vi "XY_translation_Z_rotation.vi"() -> ()   [LabVIEW 2021]
uses:
  <instrlib>/Xbox-One-Controller/Private/Type Defs/Indicators/Controller.ctl
  <instrlib>/Xbox-One-Controller/Private/Type Defs/Indicators/A.ctl
  <instrlib>/Xbox-One-Controller/Private/Type Defs/Indicators/B.ctl
  <instrlib>/Xbox-One-Controller/Private/Type Defs/Indicators/X.ctl
  <instrlib>/Xbox-One-Controller/Private/Type Defs/Indicators/Y.ctl
  <instrlib>/Xbox-One-Controller/Private/Type Defs/Indicators/Left Bumper.ctl
  <instrlib>/Xbox-One-Controller/Private/Type Defs/Indicators/Right Bumper.ctl
  <instrlib>/Xbox-One-Controller/Private/Type Defs/Indicators/View.ctl
  <instrlib>/Xbox-One-Controller/Private/Type Defs/Indicators/Menu.ctl
  <instrlib>/Xbox-One-Controller/Private/Type Defs/Indicators/Thumbstick_Analog.ctl
  <instrlib>/Xbox-One-Controller/Private/Type Defs/Indicators/Slider.ctl
  <instrlib>/Xbox-One-Controller/Private/Type Defs/Indicators/DPad.ctl
  C:/Program Files (x86)/Control/SC3U.dll
  <vilib>/Platform/TimedLoop/XDataNode/timing_clust.ctl
  <vilib>/Platform/TimedLoop/XDataNode/nitl_modes.ctl
  <vilib>/Platform/TimedLoop/XDataNode/wakeup.ctl
  <instrlib>/Xbox-One-Controller/Public/Open First Controller.vi
  <vilib>/Platform/TimedLoop/XDataNode/XDataNode.xnode
  <vilib>/Platform/TimedLoop/XDataNode/XDNodeRunTimeDep.lvlib
  <instrlib>/Xbox-One-Controller/LMH-Xbox-One-Controller.lvlib
panel:
  out "Pos X":dbl
  out "Pos Z":dbl
  in  "Com Close 3":bool
  in  "Displace Z":i64
  out "Pos Y mm":dbl
  in  "Displace Y":i64
  in  "Com Close 2":bool
  in  "Stop Button":bool
  out "Controller":T1={"A Button"=FALSE, "B Button"=FALSE, "X Button"=FALSE, "Y Button"=FALSE, "Left Bumper"=FALSE, "Right Bumper"=FALSE, "View Button"=FALSE, "Menu Button"=FALSE, "Left Stick"={[], []}, "Right Stick"={[], []}, "Trigger"=0, "D-Pad"=5} {"Trigger" scale=32767.0..-32768.0}
  in  "SC3U":refnum<k24>(container)
  in  "Com Close":bool
  in  "Displace X":i64
  out "ConnectStatus":bool
  out "ComUsing":i16
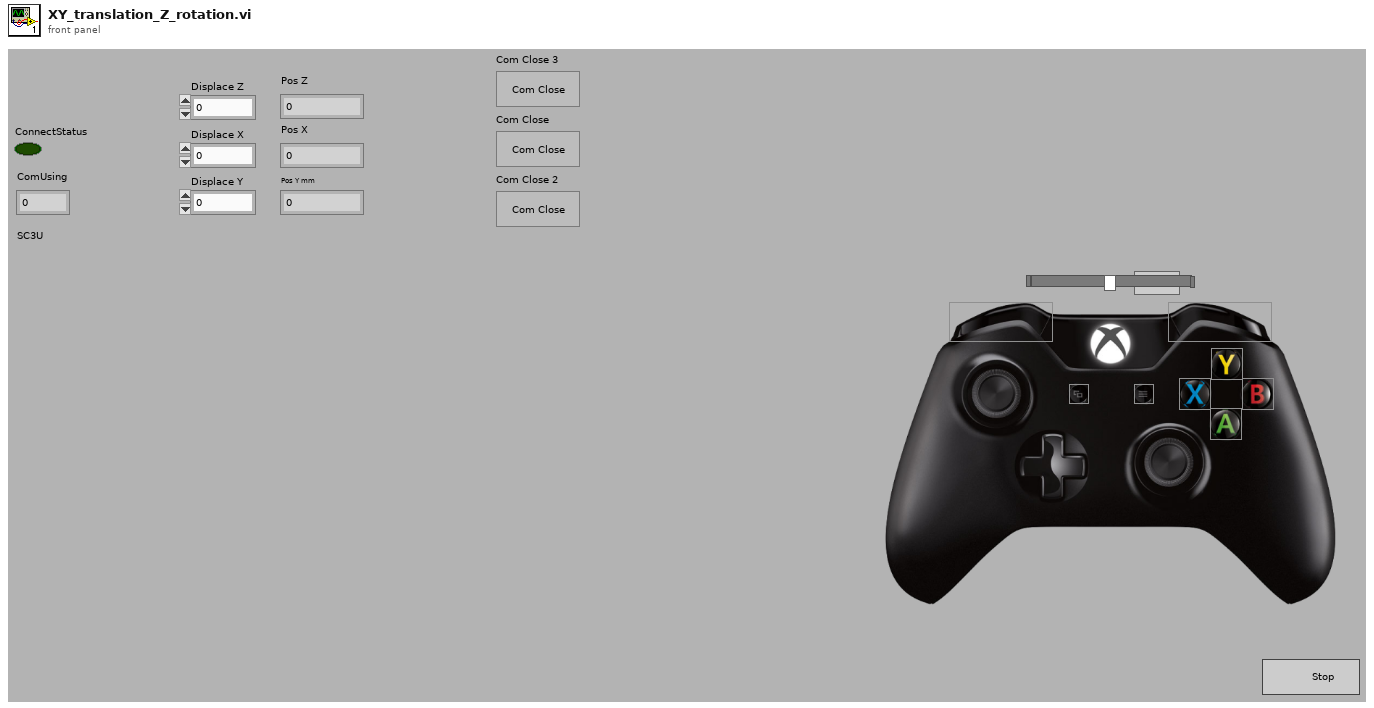
[diagram p1: front panel]
types:
  T1 = typedef "LMH-Xbox-One-Controller.lvlib/Controller.ctl" = cluster{"A Button":T2, "B Button":T3, "X Button":T4, "Y Button":T5, "Left Bumper":T6, "Right Bumper":T7, "View Button":T8, "Menu Button":T9, "Left Stick":T10, "Right Stick":T10, "Trigger":T11, "D-Pad":T12}
  T2 = typedef "LMH-Xbox-One-Controller.lvlib/A.ctl" = bool
  T3 = typedef "LMH-Xbox-One-Controller.lvlib/B.ctl" = bool
  T4 = typedef "LMH-Xbox-One-Controller.lvlib/X.ctl" = bool
  T5 = typedef "LMH-Xbox-One-Controller.lvlib/Y.ctl" = bool
  T6 = typedef "LMH-Xbox-One-Controller.lvlib/Left Bumper.ctl" = bool
  T7 = typedef "LMH-Xbox-One-Controller.lvlib/Right Bumper.ctl" = bool
  T8 = typedef "LMH-Xbox-One-Controller.lvlib/View.ctl" = bool
  T9 = typedef "LMH-Xbox-One-Controller.lvlib/Menu.ctl" = bool
  T10 = typedef "LMH-Xbox-One-Controller.lvlib/Thumbstick_Analog.ctl" = cluster{i32[], i32[]}
  T11 = typedef "LMH-Xbox-One-Controller.lvlib/Slider.ctl" = i32
  T12 = typedef "LMH-Xbox-One-Controller.lvlib/DPad.ctl" = u16
  T13 = typedef "XDNodeRunTimeDep.lvlib/timing_clust.ctl" = cluster{"Expected End [f-1]":u64, "Actual End [f-1]":u64, "Finished Late? [f-1]":bool, "Expected End [i-1]":u64, "Actual End [i-1]":u64, "Finished Late? [i-1]":bool, "Expected Start [i]":u64, "Actual Start [i]":u64, "Expected Start [f]":u64, "Actual Start [f]":u64, "Source Name":string, "Structure Name":string, "Period":i64, "Deadline":i64, "Offset":i64, "Start":i64, "Priority":i32, "Timeout":i32, "Mode":T14, "Wakeup Reason":T15, "Error":errorcluster, "Source Type":string, "Secondary Source Type":string, "Global End Time":u64, "Global Start Time":u64, "Frame Duration":u64, "Iteration Duration":u64, "Assigned CPU":i32, "I/O Scan Engine Mode":u32}
  T14 = typedef "XDNodeRunTimeDep.lvlib/nitl_modes.ctl" = enum32{"No Change", "Process missed periods, maintain original phase", "Discard missed periods, maintain original phase", "Process missed periods, ignore original phase", "Discard missed periods, ignore original phase"}
  T15 = typedef "XDNodeRunTimeDep.lvlib/wakeup.ctl" = enum32{"Normal", "Aborted", "Asynchronous wakeup", "Timing source error", "Timed loop error", "Timeout"}
  T16 = typedef "LMH-Xbox-One-Controller.lvlib/Xbox One Controller Ref.ctl" = cluster{"Controller Ref":refnum<k1>, "Event Refnum":refnum<event-registration>, "Worker Ref":refnum<vi>}
  T17 = typedef "LMH-Xbox-One-Controller.lvlib/All Axis Data.ctl" = cluster{"Left Stick":cluster{"X Axis":i32, "Y Axis":i32}, "Right Stick":cluster{"X Axis":i32, "Y Axis":i32}, "Triggers":i32, "D-Pad":T18}
  T18 = typedef "LMH-Xbox-One-Controller.lvlib/DPad Enum.ctl" = enum16{"Idle", "Up", "Up / Right", "Right", "Down / Right", "Down", "Down / Left", "Left", "Up / Left"}
  T19 = typedef "LMH-Xbox-One-Controller.lvlib/All Buttons Visual.ctl" = cluster{"A":T2, "B":T3, "X":T4, "Y":T5, "Left Bumper":T6, "Right Bumper":T7, "View Button":T8, "Menu Button":T9, "Left Stick":T20, "Right Stick":T20}
  T20 = typedef "LMH-Xbox-One-Controller.lvlib/Thumbstick.ctl" = bool
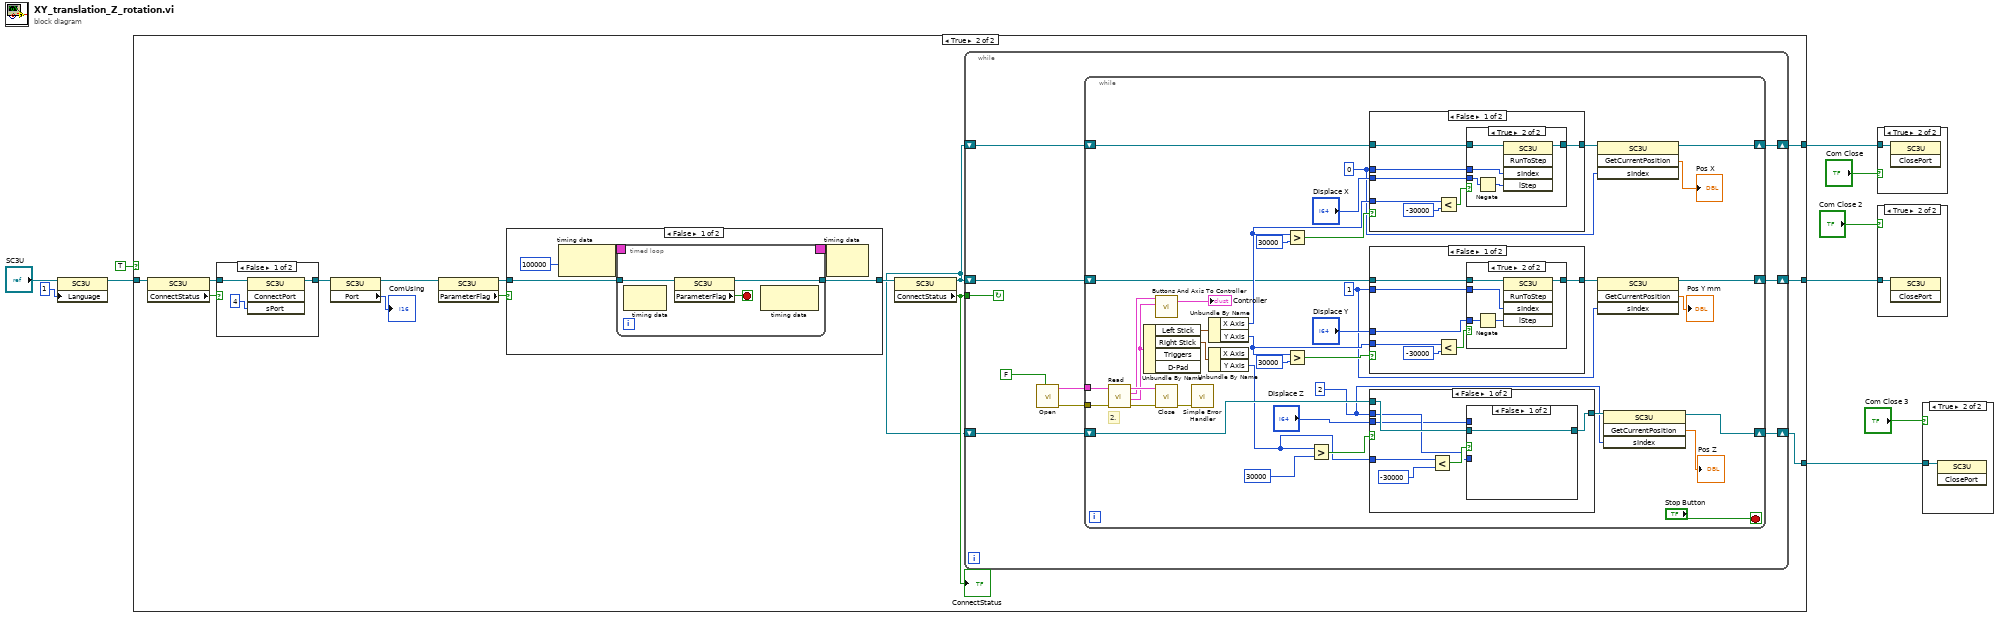
[diagram p0: block diagram]
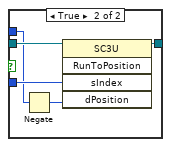
[diagram p6: hidden frame]
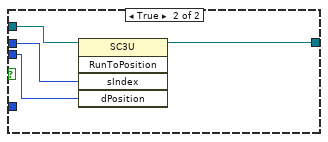
[diagram p7: hidden frame]
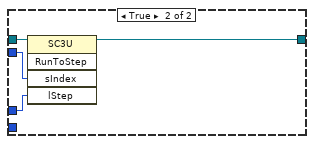
[diagram p9: hidden frame]
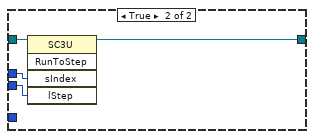
[diagram p11: hidden frame]
diagram:
  n1 = property class="SC3U"(reference="SC3U", "Language"=i16 1 ("intLanguage")) -> (reference out=w3:refnum<k24>)  [unwired: 1 in, 1 out]
  n2 = case shown="True" TRUE {
    tunnel: [_ w14] -> w6
    tunnel: w3 -> [_ w23]
    tunnel: [_ w13] -> w4
    tunnel: [_ w11] -> w1
    frame False {
    }
    frame True {
      n3 = property class="SC3U"(reference=w23) -> (reference out=w22:refnum<k24>, "ConnectStatus"=w21:bool)  [unwired: 1 in, 1 out]
      n4 = case shown="False" w21 {
        tunnel: w22 -> [w141 w142]
        tunnel: [w140 w142] -> w20
        frame False {
          n5 = invoke class="SC3U" method="ConnectPort"(reference=w141, "sPort"=i16 4 ("ComUsing")) -> (reference out=w140:refnum<k24>)  [unwired: 2 in, 3 out]
        }
        frame True {
        }
      }
      n6 = property class="SC3U"(reference=w20) -> (reference out=w18:refnum<k24>, "Port"=→"ComUsing":i16)  [unwired: 1 in, 1 out]
      n7 = property class="SC3U"(reference=w18) -> (reference out=w17:refnum<k24>, "ParameterFlag"=w16:bool)  [unwired: 1 in, 1 out]
      n8 = case shown="False" w16 {
        tunnel: w17 -> [w125 w138]
        tunnel: [w124 w138] -> w24
        frame False {
          n9 = node-c288(i64 100000 ("周期")) -> (w128:T13)
          n10 = timed-loop {
            timing: w128 -> [_]
            timing-out: [_] -> w127
            tunnel: w125 -> [w131]
            tunnel: [w130] -> w124
            stop <- w129 stop-if-true
            n11 = node-c288() -> ()  [unwired: 1 in, 1 out]
            n12 = property class="SC3U"(reference=w131) -> (reference out=w130:refnum<k24>, "ParameterFlag"=w129:bool)  [unwired: 1 in, 1 out]
            n13 = node-c288() -> ()  [unwired: 1 in, 1 out]
          }
          n14 = node-c288(w127) -> ()  [unwired: 1 out]
        }
        frame True {
        }
      }
      n15 = property class="SC3U"(reference=w24) -> (reference out=w12:refnum<k24>, "ConnectStatus"=w15:bool)  [unwired: 1 in, 1 out]
      "ConnectStatus" <- w15
      n16 = while {
        shift-right: [w34] -> w14
        shift-left: w12 -> [w33]
        tunnel: w15 -> [w32]
        shift-right: [w27] -> w13
        shift-left: w12 -> [w28]
        shift-right: [w25] -> w11
        shift-left: w12 -> [w26]
        stop <- w32 continue-if-true
        n17 = call-poly <instrlib>:"Open.vi"("Enable Events (T)"=FALSE) -> ("Error Out"=w30:errorcluster, "Xbox One Controller"=w31:T16)  [unwired: 8 in, 1 out]
        n18 = while {
          tunnel: w31 -> [w69]
          tunnel: w30 -> [w68]
          shift-right: [w51] -> w34
          shift-left: w33 -> [w72]
          shift-right: [w48] -> w27
          shift-left: w28 -> [w54]
          shift-right: [w39] -> w25
          shift-left: w26 -> [w40]
          stop <- "Stop Button" stop-if-true
          w38 = 2
          w46 = 1
          w50 = 0
          # "2."
          n19 = call <instrlib>:"Read.vi"("Error In"=w68, "Xbox One Controller Ref"=w69) -> ("Error Out"=w66:errorcluster, "All Axis"=w64:T17, "Buttons"=w58:T19, "Xbox One Controller Ref"=w65:T16)  [unwired: 6 in]
          n20 = Unbundle By Name(w64) -> ("Left Stick"=w71:cluster{"X Axis":i32, "Y Axis":i32}, "Right Stick"=w37:cluster{"X Axis":i32, "Y Axis":i32})  [unwired: 2 out]
          n21 = call <instrlib>:"Buttons And Axis To Controller.vi"("All Axis"=w64, "Buttons"=w58) -> ("Controller"=→"Controller":T1)  [unwired: 5 in]
          n22 = call <instrlib>:"Close.vi"("Error In"=w66, "Xbox One Controller Ref"=w65) -> ("Error Out"=w67:errorcluster)  [unwired: 9 in]
          n23 = call <vilib>:"Simple Error Handler.vi"("error in (no error)"=w67) -> ()  [unwired: 4 in, 5 out]
          n24 = Unbundle By Name(w71) -> ("X Axis"=w60:i32, "Y Axis"=w53:i32)
          n25 = Unbundle By Name(w37) -> ("Y Axis"=w36:i32)  [unwired: 1 out]
          n26 = Greater?(x=w60, y=30000) -> (0:w61:bool)
          n27 = Greater?(x=w53, y=30000) -> (0:w56:bool)
          n28 = Greater?(x=w36, y=30000) -> (0:w44:bool)
          n29 = case shown="False" w44 {
            tunnel: w38 -> [w74 w89]
            tunnel: "Displace Z" -> [w73 w88]
            tunnel: w40 -> [w76 w87]
            tunnel: [w75 w86] -> w42
            tunnel: w36 -> [w79 _]
            frame False {
              n30 = Less?(x=w79, y=-30000) -> (x < y?=w77:bool)
              n31 = case shown="False" w77 {
                tunnel: w76 -> [w80 w85]
                tunnel: [w80 w84] -> w75
                tunnel: w74 -> [_ w83]
                tunnel: w73 -> [_ w81]
                frame False {
                }
                frame True {
                  n32 = Negate(x=w81) -> (-x=w82:i64)
                  n33 = invoke class="SC3U" method="RunToPosition"(reference=w85, "sIndex"=w83, "dPosition"=w82) -> (reference out=w84:refnum<k24>)  [unwired: 2 in, 4 out]
                }
              }
            }
            frame True {
              n34 = invoke class="SC3U" method="RunToPosition"(reference=w87, "sIndex"=w89, "dPosition"=w88) -> (reference out=w86:refnum<k24>)  [unwired: 2 in, 4 out]
            }
          }
          n35 = case shown="False" w61 {
            tunnel: [w112 w120] -> w52
            tunnel: w72 -> [w113 w123]
            tunnel: w60 -> [w111 _]
            tunnel: "Displace X" -> [w108 w122]
            tunnel: w50 -> [w107 w121]
            frame False {
              n36 = Less?(x=w111, y=-30000) -> (x < y?=w109:bool)
              n37 = case shown="True" w109 {
                tunnel: w113 -> [w114 w119]
                tunnel: [w114 w115] -> w112
                tunnel: w108 -> [_ w117]
                tunnel: w107 -> [_ w116]
                frame False {
                }
                frame True {
                  n38 = Negate(x=w117) -> (-x=w118:i64)
                  n39 = invoke class="SC3U" method="RunToStep"(reference=w119, "sIndex"=w116, "lStep"=w118) -> (reference out=w115:refnum<k24>)  [unwired: 2 in, 4 out]
                }
              }
            }
            frame True {
              n40 = invoke class="SC3U" method="RunToStep"(reference=w123, "sIndex"=w121, "lStep"=w122) -> (reference out=w120:refnum<k24>)  [unwired: 2 in, 4 out]
            }
          }
          n41 = case shown="False" w56 {
            tunnel: [w95 w103] -> w49
            tunnel: w54 -> [w96 w106]
            tunnel: w53 -> [w94 _]
            tunnel: "Displace Y" -> [w90 w105]
            tunnel: w46 -> [w91 w104]
            frame False {
              n42 = Less?(x=w94, y=-30000) -> (x < y?=w92:bool)
              n43 = case shown="True" w92 {
                tunnel: w96 -> [w97 w102]
                tunnel: [w97 w98] -> w95
                tunnel: w90 -> [_ w100]
                tunnel: w91 -> [_ w99]
                frame False {
                }
                frame True {
                  n44 = Negate(x=w100) -> (-x=w101:i64)
                  n45 = invoke class="SC3U" method="RunToStep"(reference=w102, "sIndex"=w99, "lStep"=w101) -> (reference out=w98:refnum<k24>)  [unwired: 2 in, 4 out]
                }
              }
            }
            frame True {
              n46 = invoke class="SC3U" method="RunToStep"(reference=w106, "sIndex"=w104, "lStep"=w105) -> (reference out=w103:refnum<k24>)  [unwired: 2 in, 4 out]
            }
          }
          n47 = invoke class="SC3U" method="GetCurrentPosition"(reference=w52, "sIndex"=w50) -> (reference out=w51:refnum<k24>, "GetCurrentPosition"=→"Pos X":dbl)  [unwired: 2 in, 2 out]
          n48 = invoke class="SC3U" method="GetCurrentPosition"(reference=w49, "sIndex"=w46) -> (reference out=w48:refnum<k24>, "GetCurrentPosition"=→"Pos Y mm":dbl)  [unwired: 2 in, 2 out]
          n49 = invoke class="SC3U" method="GetCurrentPosition"(reference=w42, "sIndex"=w38) -> (reference out=w39:refnum<k24>, "GetCurrentPosition"=→"Pos Z":dbl)  [unwired: 2 in, 2 out]
        }
      }
    }
  }
  n50 = case shown="True" "Com Close" {
    tunnel: w6 -> [_ w143]
    frame False {
    }
    frame True {
      n51 = invoke class="SC3U" method="ClosePort"(reference=w143) -> ()  [unwired: 2 in, 3 out]
    }
  }
  n52 = case shown="True" "Com Close 2" {
    tunnel: w4 -> [_ w144]
    frame False {
    }
    frame True {
      n53 = invoke class="SC3U" method="ClosePort"(reference=w144) -> ()  [unwired: 2 in, 3 out]
    }
  }
  n54 = case shown="True" "Com Close 3" {
    tunnel: w1 -> [_ w145]
    frame False {
    }
    frame True {
      n55 = invoke class="SC3U" method="ClosePort"(reference=w145) -> ()  [unwired: 2 in, 3 out]
    }
  }
